vi "Set Queue Attributes.vi"(8 "error in (no error)":errorcluster, 10 "Attributes":T1[](array[typedef]), 11 "SQS in":refnum<class "SQS.lvclass">) -> (0 "error out":errorcluster, 3 "SQS out":refnum<class "SQS.lvclass">)   [LabVIEW 2015, in "NI_SQS.lvlib" / "SQS.lvclass"]
uses:
  SQS.lvclass
  Attribute Value Pair.ctl
  Queue Attribute.ctl
  Core/Name Value Pair.ctl
  Core/Request Options.ctl
  SQS.lvclass/SQS.ctl
  Read Account Number.vi
  Read Name.vi
  Core/NI_AWS Core.lvlib
  NI_SQS.lvlib
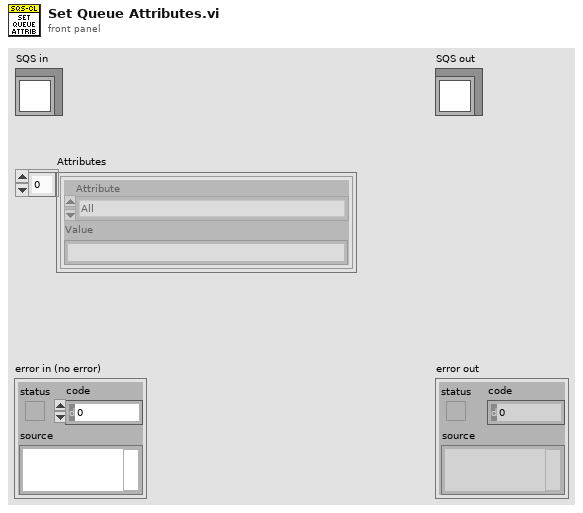
[diagram p1: front panel]
types:
  T1 = typedef "NI_SQS.lvlib/Attribute Value Pair.ctl" = cluster{"Attribute":T2, "Value":string}
  T2 = typedef "NI_SQS.lvlib/Queue Attribute.ctl" = enum16{"All", "Policy", "VisibilityTimeout", "MaximumMessageSize", "MessageRetentionPeriod", "ApproximateNumberOfMessages", "ApproximateNumberOfMessagesNotVisible", "CreatedTimestamp", "LastModifiedTimestamp", "QueueArn", "ApproximateNumberOfMessagesDelayed", "DelaySeconds", "ReceiveMessageWaitTimeSeconds", "RedrivePolicy", "FifoQueue", "ContentBasedDeduplication"}
  T3 = typedef "NI_AWS Core.lvlib/Request Options.ctl" = cluster{"request headers":T4[], "request parameters":T4[], "request body":string}
  T4 = typedef "NI_AWS Core.lvlib/Name Value Pair.ctl" = cluster{"name":string, "value":string}
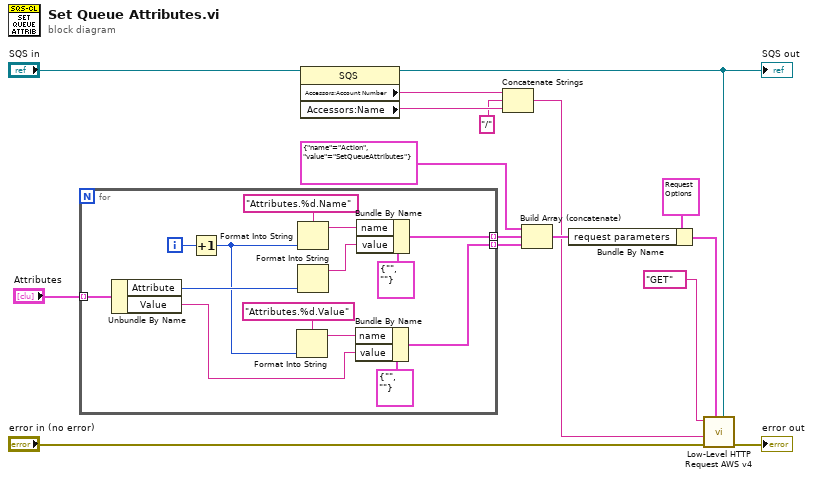
[diagram p0: block diagram]
diagram:
  n1 = for {
    tunnel: "Attributes" -> [w25] mode=indexing
    tunnel: [w26] -> w8 mode=indexing
    tunnel: [w19] -> w1 mode=indexing
    i -> [w30]
    n2 = Unbundle By Name(w25) -> ("Attribute"=w23:T2, "Value"=w17:string)
    n3 = Increment(x=w30) -> (x+1=w18:i32)
    n4 = Format Into String(format string="Attributes.%d.Value", w18) -> (resulting string=w22:string)  [unwired: 2 in, 1 out]
    n5 = Format Into String(format string="Attributes.%d.Name", w18) -> (resulting string=w27:string)  [unwired: 2 in, 1 out]
    n6 = Format Into String(w23) -> (resulting string=w24:string)  [unwired: 3 in, 1 out]
    n7 = Bundle By Name(cluster=T4 {"name"="", "value"=""} ("element"), "name"=w22, "value"=w17) -> (w19:T4)
    n8 = Bundle By Name(cluster=T4 {"name"="", "value"=""} ("element"), "name"=w27, "value"=w24) -> (w26:T4)
  }
  n9 = property class="SQS"(reference="SQS in") -> (reference out=w7:refnum<class "SQS.lvclass">, "Accessors:Account Number"=w6:string, "Accessors:Name"=w5:string)  [unwired: 1 in, 1 out]
  "SQS out" <- w7
  n10 = Concatenate Strings(w6, "/", w5) -> (w3:string)
  n11 = Build Array (concatenate)(T4 {"name"="Action", "value"="SetQueueAttributes"} ("Cluster"), w8, w1) -> (w9:T4[])
  n12 = Bundle By Name(cluster=T3 {"request headers"=[], "request parameters"=[{"name"="Action", "value"="ListQueues"}], "request body"=""} ("Request Options"), "request parameters"=w9) -> (w10:T3)
  n13 = call "Low-Level HTTP Request AWS v4.vi"("AWS Core"=w7, "Request Options"=w10, "error in (no error)"="error in (no error)", "URL Suffix"=w3, "HTTP-Verb"="GET") -> ("error out"=→"error out":errorcluster)  [unwired: 4 in, 2 out]
